vi "DataLock.vi"() -> ()   [LabVIEW 2019, in "Global.lvlib"]
uses:
  Global.lvlib
panel:
  out "Lock":bool
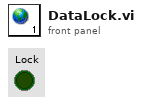
[diagram p1: front panel]
diagram:
